vi "Get Default Property.vi"(11 "Index":i32) -> (3 "Temporary Property":T1)   [LabVIEW 2020, in "2D Feather.lvclass"]
uses:
  <vilib>/Math Plots/2D Math Plots/2D Feather/2D Feather/2D Feather.lvclass
  <vilib>/Math Plots/2D Math Plots/2D Plot/2D Plot/Typedef/Plot Property.ctl
  <vilib>/Math Plots/2D Math Plots/2D Plot/2D Plot/2D Plot.lvclass
panel:
  in  "Plot Prefix":string="Plot "
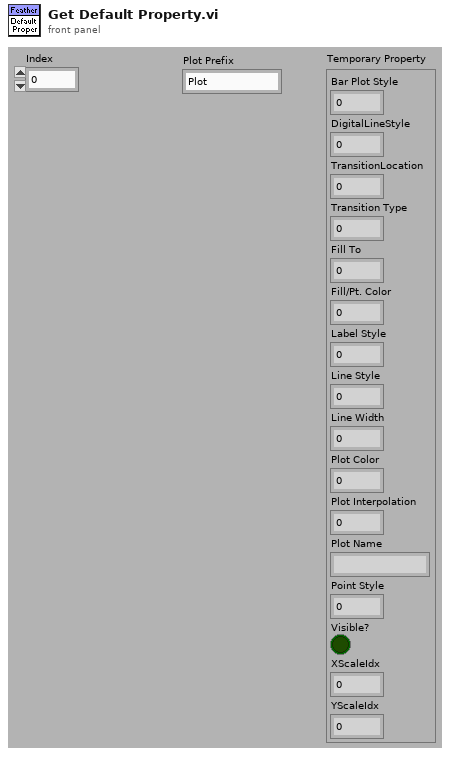
[diagram p1: front panel]
types:
  T1 = typedef "2D Plot.lvclass/Plot Property.ctl" = cluster{"Bar Plot Style":u8, "DigitalLineStyle":u8, "TransitionLocation":u8, "Transition Type":u8, "Fill To":i16, "Fill/Pt. Color":u32, "Label Style":u8, "Line Style":u8, "Line Width":u8, "Plot Color":u32, "Plot Interpolation":u8, "Plot Name":string, "Point Style":u8, "Visible?":bool, "XScaleIdx":u32, "YScaleIdx":u32}
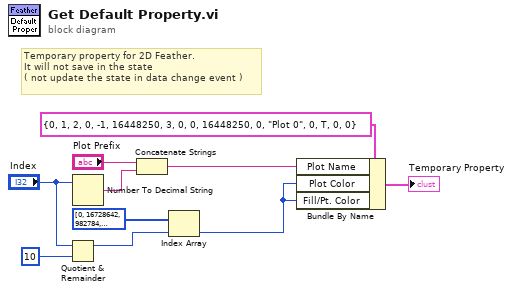
[diagram p0: block diagram]
diagram:
  # "Temporary property for 2D Feather.\nIt will not save in the state\n( not update the state in data change event )"
  n1 = Quotient & Remainder(x="Index", y=10) -> (x-y*floor(x/y)=w5:i32)  [unwired: 1 out]
  n2 = Number To Decimal String(number="Index") -> (decimal integer string=w9:string)  [unwired: 1 out]
  n3 = Concatenate Strings("Plot Prefix", w9) -> (w8:string)
  n4 = Index Array(array=u32[] [0, 16728642, 982784, 4375295, 13827953, 13457919, 16757522, 4343295, 16728758, 5898228] ("Array"), index=w5) -> (element=w1:u32)
  n5 = Bundle By Name(cluster=T1 {"Bar Plot Style"=0, "DigitalLineStyle"=1, "TransitionLocation"=2, "Transition Type"=0, "Fill To"=-1, "Fill/Pt. Color"=16448250, "Label Style"=3, "Line Style"=0, "Line Width"=0, "Plot Color"=16448250, "Plot Interpolation"=0, "Plot Name"="Plot 0", "Point Style"=0, "Visible?"=TRUE, "XScaleIdx"=0, "YScaleIdx"=0} ("Plot Property"), "Plot Name"=w8, "Plot Color"=w1, "Fill/Pt. Color"=w1) -> (→"Temporary Property":T1)
